vi "CRYVariable Correspond Table.vi"(11 "Variables In":string[](array[string])) -> (1 "Correspond Table":string[][](array[string]), 3 "New Variables":string[](array[string]))   [LabVIEW 2013]
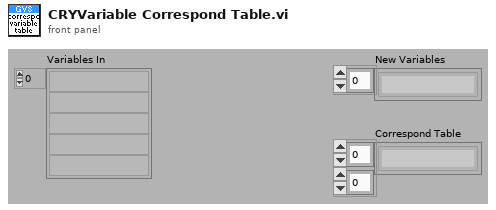
[diagram p1: front panel]
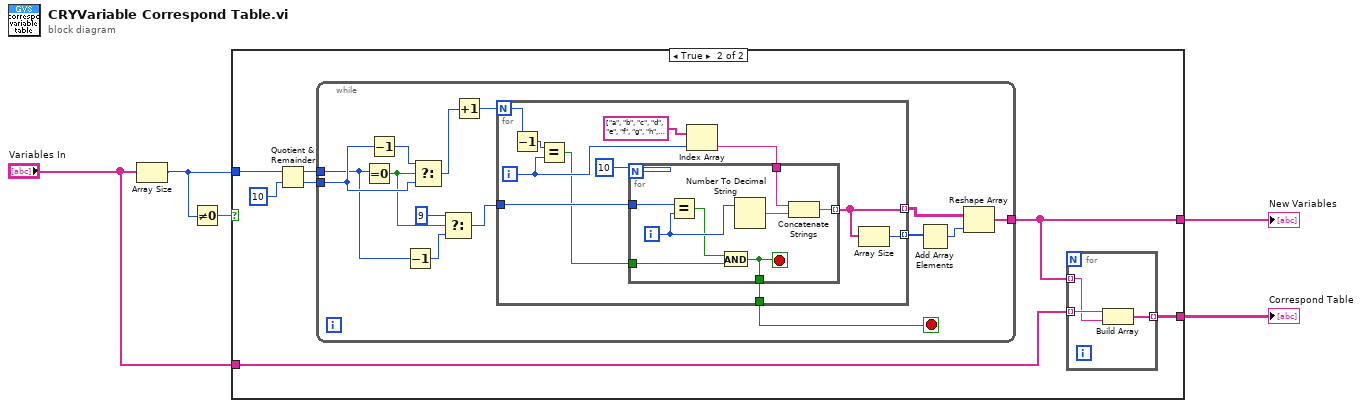
[diagram p0: block diagram]
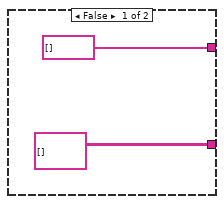
[diagram p2: hidden frame]
diagram:
  n1 = Array Size(array="Variables In") -> (size(s)=w1:i32)
  n2 = Not Equal To 0?(x=w1) -> (x != 0?=w5:bool)
  n3 = case shown="True" w5 {
    tunnel: w1 -> [_ w11]
    tunnel: [string[] [] w9] -> w4
    tunnel: "Variables In" -> [_ w10]
    tunnel: [string[][] [] w8] -> w2
    frame False {
    }
    frame True {
      n4 = Quotient & Remainder(x=w11, y=10) -> (x-y*floor(x/y)=w12:i32, floor(x/y)=w13:i32)
      n5 = while {
        tunnel: w13 -> [w31]
        tunnel: w12 -> [w30]
        tunnel: [w18] -> w9
        stop <- w26 stop-if-true
        n6 = Equal To 0?(x=w30) -> (x = 0?=w25:bool)
        n7 = Decrement(x=w31) -> (x-1=w29:i32)
        n8 = Decrement(x=w30) -> (x-1=w24:i32)
        n9 = Select(t=w29, s=w25, f=w31) -> (s? t:f=w28:i32)
        n10 = Select(t=9, s=w25, f=w24) -> (s? t:f=w22:i32)
        n11 = Increment(x=w28) -> (x+1=w27:i32)
        n12 = for {
          N: w27 -> [w38]
          tunnel: [w33] -> w19 mode=indexing
          tunnel: w22 -> [w36]
          tunnel: [w34] -> w26
          tunnel: [w32] -> w21 mode=indexing
          i -> [w39]
          n13 = Decrement(x=w38) -> (x-1=w37:i32)
          n14 = Equal?(x=w37, y=w39) -> (x = y?=w35:bool)
          n15 = Index Array(array=string[] ["a", "b", "c", "d", "e", "f", "g", "h", "i", "j", "k", "l", "m", "n", "o", "p", "q", "r", "s", "t", "u", "v", "w", "x", "y", "z"] ("Variables Out"), index=w39) -> (element=w40:string)
          n16 = for {
            N: 10 -> [_]
            tunnel: w40 -> [w49]
            tunnel: [w48] -> w33 mode=indexing
            tunnel: w36 -> [w47]
            tunnel: w35 -> [w44]
            tunnel: [w43] -> w34
            i -> [w46]
            stop <- w43 stop-if-true
            n17 = Equal?(x=w47, y=w46) -> (x = y?=w45:bool)
            n18 = And(x=w45, y=w44) -> (x .and. y?=w43:bool)
            n19 = Number To Decimal String(number=w46) -> (decimal integer string=w50:string)  [unwired: 1 in]
            n20 = Concatenate Strings(w49, w50) -> (w48:string)
          }
          n21 = Array Size(array=w33) -> (size(s)=w32:i32)
        }
        n22 = Add Array Elements(numeric array=w21) -> (sum=w20:i32)
        n23 = Reshape Array(w19, w20) -> (w18:string[])
      }
      n24 = for {
        tunnel: w10 -> [w17] mode=indexing
        tunnel: w9 -> [w16] mode=indexing
        tunnel: [w15] -> w8 mode=indexing
        n25 = Build Array(w17, w16) -> (w15:string[])
      }
    }
  }
  "New Variables" <- w4
  "Correspond Table" <- w2
